vi "File.Folder to Zip File.vi"(8 "error in (no error)":errorcluster, 9 "Output Folder":path, 11 "Source Folder":path) -> (0 "error out":errorcluster, 1 "Duration(s)":dbl, 3 "Zip File":path)   [LabVIEW 2018]
uses:
  <vilib>/KATE/Time/Time Utils.lvlib
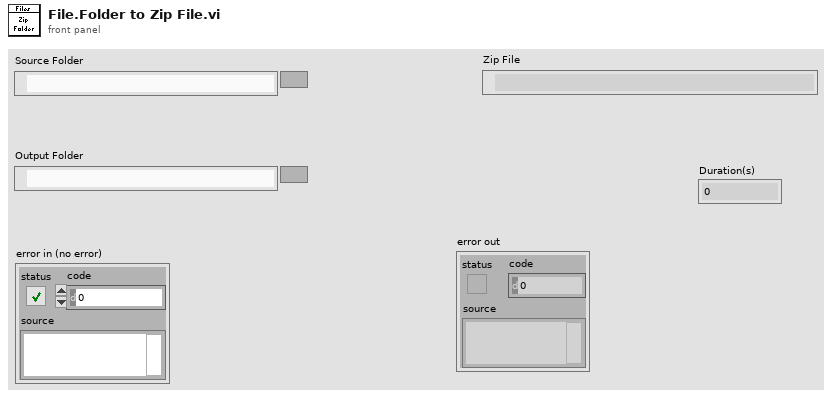
[diagram p1: front panel]
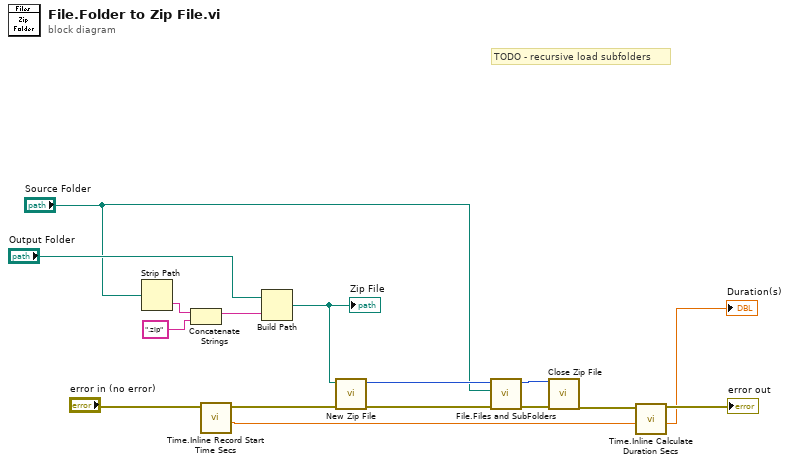
[diagram p0: block diagram]
diagram:
  # "TODO - recursive load subfolders"
  n1 = Strip Path(path="Source Folder") -> (name=w16:string)  [unwired: 1 out]
  n2 = Concatenate Strings(w16, ".zip") -> (w14:string)
  n3 = call <vilib>:"Time.Inline Record Start Time Secs.vi"("Error In Upper"="error in (no error)") -> ("Start(s)"=w7:dbl, "Error Out Upper"=w8:errorcluster)  [unwired: 8 in, 1 out]
  n4 = Build Path(base path="Output Folder", name or relative path=w14) -> (appended path=w12:path)
  "Zip File" <- w12
  n5 = call <vilib>:"New Zip File.vi"("error in (no error)"=w8, "target"=w12) -> ("error out"=w4:errorcluster, "zip file out"=w5:i64)  [unwired: 3 in, 1 out]
  n6 = call "File.Files and SubFolders.vi"("error in"=w4, "Folder"="Source Folder", "Zip File"=w5) -> ("error out"=w1:errorcluster, "Zip File Out"=w2:i64)  [unwired: 6 in, 1 out]
  n7 = call <vilib>:"Close Zip File.vi"("error in (no error)"=w1, "zip file in"=w2) -> ("error out"=w11:errorcluster)  [unwired: 5 in]
  n8 = call <vilib>:"Time.Inline Calculate Duration Secs.vi"("Start(Sec)"=w7, "Error In Top"=w11) -> ("Duration(s)"=→"Duration(s)":dbl, "Error Out Top"=→"error out":errorcluster)  [unwired: 7 in, 1 out]
